vi "JKI Get System Web Browser__jki_lib_communication -- VI Tester.vi"(4 "error in (no error)":errorcluster) -> (0 "error out":errorcluster, 3 "browser command":string)   [LabVIEW 2011]
uses:
  <vilib>/registry/registry.llb/Registry RtKey.ctl
  <vilib>/registry/registry.llb/Read Registry Value Simple STR.vi
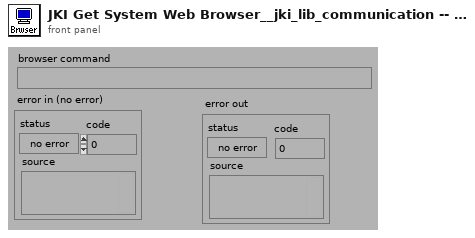
[diagram p1: front panel]
types:
  T1 = enum32{"KEY_QUERY_VALUE", "KEY_SET_VALUE", "KEY_CREATE_SUB_KEY", "KEY_ENUMERATE_SUB_KEYS", "KEY_NOTIFY", "KEY_CREATE_LINK", "KEY_READ", "KEY_WRITE", "KEY_ALL_ACCESS", "KEY_READ | KEY_WRITE"}
  T2 = typedef "Registry RtKey.ctl" = enum32{"HKEY_CLASSES_ROOT", "HKEY_CURRENT_USER", "HKEY_LOCAL_MACHINE", "HKEY_USERS", "HKEY_PERFORMANCE_DATA", "HKEY_CURRENT_CONFIG", "HKEY_DYN_DATA"}
  T3 = typedef "Registry refnum.ctl" = refnum<k1>
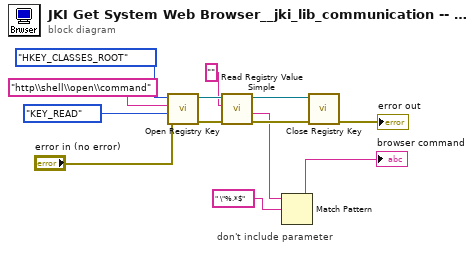
[diagram p0: block diagram]
diagram:
  # "don't include parameter"
  n1 = call <vilib>:"Open Registry Key.vi"("error in (no error)"="error in (no error)", "security access mask (KEY_READ | KEY_WRITE)"=T1."KEY_READ", "subkey"="http\\shell\\open\\command", "root key (HKEY_LOCAL_MACHINE)"=Registry_RtKey."HKEY_CLASSES_ROOT") -> ("error out"=w10:errorcluster, "refnum out"=w13:T3)  [unwired: 6 in]
  n2 = call-poly <vilib>:"Read Registry Value Simple.vi"("error in (no error)"=w10, "value"="" ("lpValueName"), "refnum"=w13) -> ("error out"=w9:errorcluster, "String/Binary data"=w5:string, "refnum out"=w3:T3)  [unwired: 3 in, 1 out]
  n3 = Match Pattern(string=w5, regular expression=" \"%.*$") -> (before substring=→"browser command":string)  [unwired: 1 in, 3 out]
  n4 = call <vilib>:"Close Registry Key.vi"("error in (no error)"=w9, "refnum"=w3) -> ("error out"=→"error out":errorcluster)  [unwired: 5 in]
